vi "Create_DO_Signal.vi"(8 "error in":errorcluster, 10 "Pre-Activation?":bool, 11 "On/Off":bool) -> (0 "error out":errorcluster, 2 "Samples":u32, 3 "WF":u32[](array[numeric]))   [LabVIEW 2021]
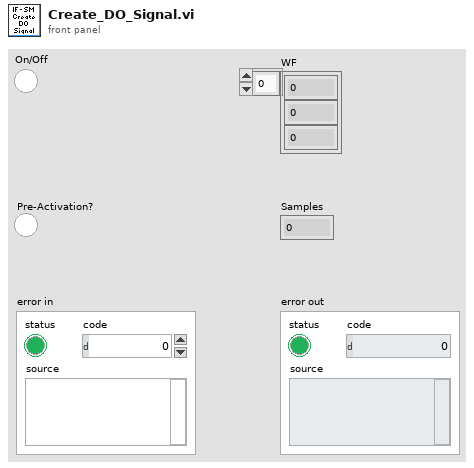
[diagram p1: front panel]
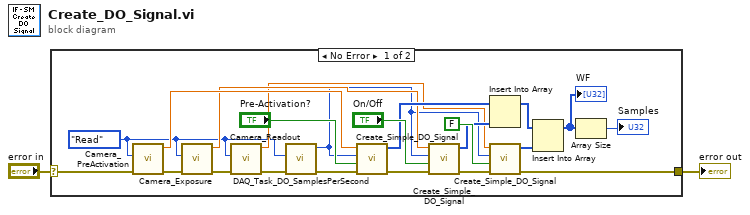
[diagram p0: block diagram]
diagram:
  n1 = case shown="No Error" "error in" {
    selector: "error in" -> [w12 w25]
    tunnel: [w3 w25] -> w1
    frame No Error {
      w7 = enum16{"Write", "Read"}."Read" ("Action")
      n2 = call "Camera_PreActivation.vi"("error in"=w12, "Action"=w7) -> ("error out"=w11:errorcluster, "Camera_PreActivation"=w13:dbl)  [unwired: 8 in]
      n3 = call "Camera_Exposure.vi"("error in"=w11, "Action"=w7) -> ("error out"=w9:errorcluster, "Exposure (s)"=w10:dbl)  [unwired: 8 in]
      n4 = call "Camera_Readout.vi"("error in"=w9, "Action"=w7) -> ("error out"=w6:errorcluster, "Camera_Readout"=w8:dbl)  [unwired: 8 in]
      n5 = call "DAQ_Task_DO_SamplesPerSecond.vi"("error in"=w6, "Action"=w7) -> ("error out"=w4:errorcluster, "DO_Task_SamplesPerSec"=w5:u32)  [unwired: 8 in]
      n6 = call "Create_Simple_DO_Signal.vi"("error in"=w4, "On/Off"="Pre-Activation?", "Samples / s (10000)"=w5, "Time (s)"=w13) -> ("error out"=w16:errorcluster, "Signal"=w14:u32[])  [unwired: 6 in]
      n7 = call "Create_Simple_DO_Signal.vi"("error in"=w16, "On/Off"="On/Off", "Samples / s (10000)"=w5, "Time (s)"=w10) -> ("error out"=w18:errorcluster, "Signal"=w17:u32[])  [unwired: 6 in]
      n8 = Insert Into Array(array=w14, new element=w17) -> (w19:u32[])  [unwired: 1 in]
      n9 = call "Create_Simple_DO_Signal.vi"("error in"=w18, "On/Off"=FALSE, "Samples / s (10000)"=w5, "Time (s)"=w8) -> ("error out"=w3:errorcluster, "Signal"=w21:u32[])  [unwired: 6 in]
      n10 = Insert Into Array(array=w19, new element=w21) -> (w20:u32[])  [unwired: 1 in]
      "WF" <- w20
      n11 = Array Size(array=w20) -> (size(s)=→"Samples":i32)
    }
    frame Error {
    }
  }
  "error out" <- w1
